vi "SaveImage.vi"(1 "error in (no error)":errorcluster, 2 "Path":path, 3 "Image Src":T1) -> (0 "error out":errorcluster)   [LabVIEW 2013, in "GxLVlib.lvlib"]
uses:
  GxLVlib.lvlib
  <vilib>/vision/Image Controls.llb/IMAQ Image.ctl
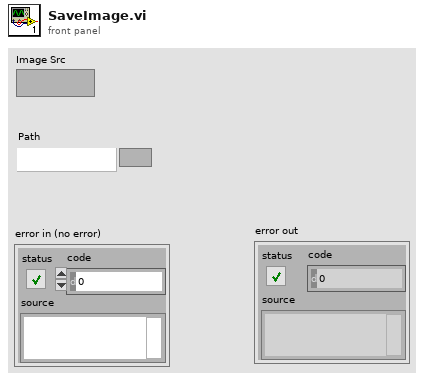
[diagram p1: front panel]
types:
  T1 = typedef "IMAQ Image.ctl" = refnum<image>
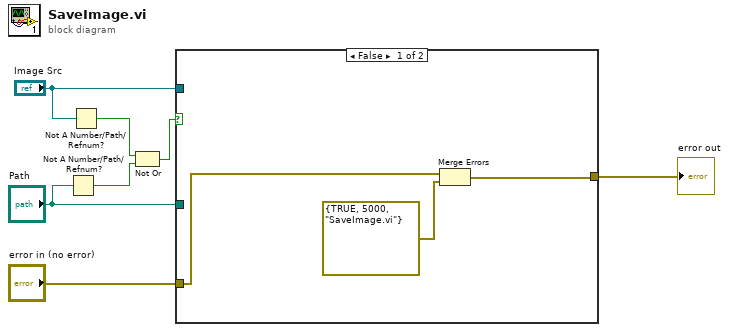
[diagram p0: block diagram]
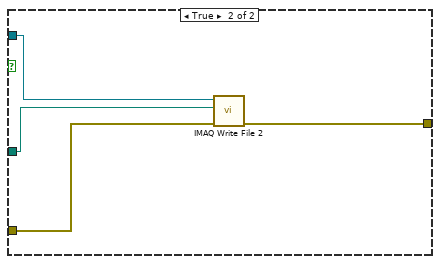
[diagram p2: hidden frame]
diagram:
  n1 = Not A Number/Path/Refnum?(number/path/refnum="Path") -> (NaN/Path/Refnum?=w6:bool)
  n2 = Not A Number/Path/Refnum?(number/path/refnum="Image Src") -> (NaN/Path/Refnum?=w7:bool)
  n3 = Not Or(1:w6, 2:w7) -> (0:w5:bool)
  n4 = case shown="False" w5 {
    tunnel: "Image Src" -> [_ w14]
    tunnel: "Path" -> [_ w13]
    tunnel: "error in (no error)" -> [w9 w12]
    tunnel: [w8 w11] -> w1
    frame False {
      n5 = Merge Errors(w9, errorcluster {TRUE, 5000, "SaveImage.vi"}) -> (w8:errorcluster)
    }
    frame True {
      n6 = call-poly "IMAQ Write File 2"("error in (no error)"=w12, "File Path"=w13, "Image"=w14) -> ("error out"=w11:errorcluster)  [unwired: 7 in, 1 out]
    }
  }
  "error out" <- w1
